vi "rqcAlice Cascade (Low Level Example).vi"() -> ()   [LabVIEW 2019]
panel:
  out "?":T1
  in  "QBER":dbl
  in  "Raw Alice's key path":string
  in  "Bob's port":string
  in  "Bob's IP":string
  out "pyton script path":path=path "../python_scripts/cascade_alice.py"
  in  "error in":errorcluster
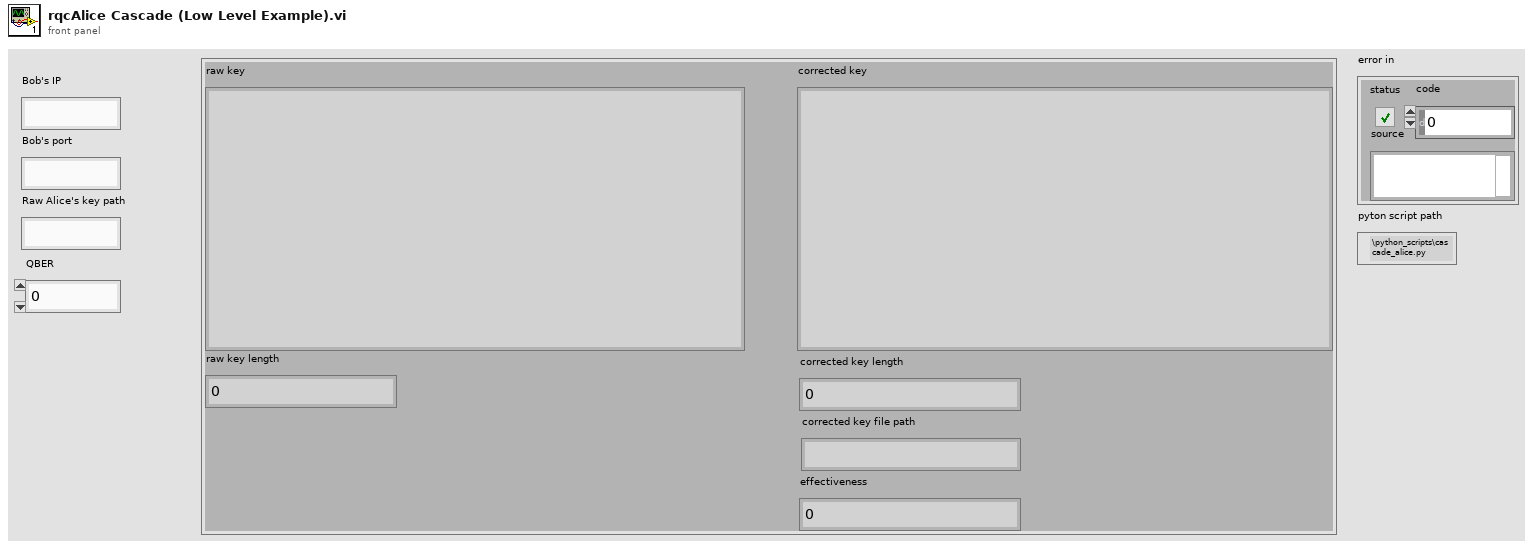
[diagram p1: front panel]
types:
  T1 = cluster{"raw key length":i32, "corrected key":string, "corrected key file path":string, "corrected key length":i32, "effectiveness":dbl, "raw key":string}
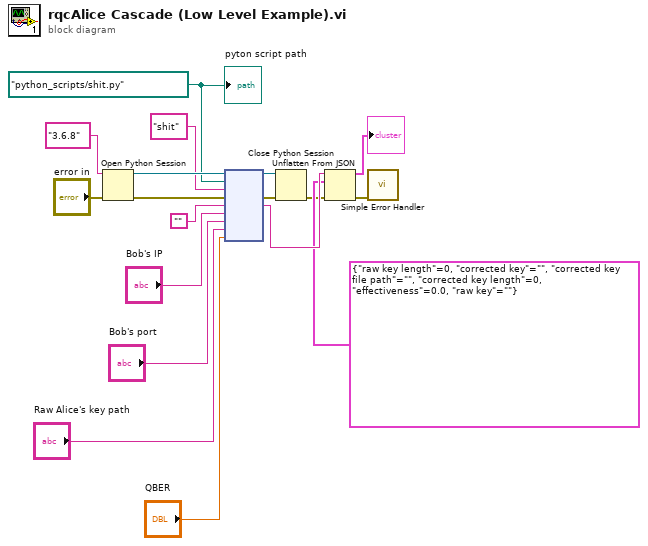
[diagram p0: block diagram]
diagram:
  w12 = path "python_scripts/shit.py" ("module path")
  n1 = Open Python Session(python version="3.6.8" ("Python version"), 3:"error in") -> (session out=w16:refnum<k35>, error out=w15:errorcluster)  [unwired: 1 in]
  n2 = node(w16, w12, "shit" ("function name"), w15, "", "Bob's IP", "Bob's port", "Raw Alice's key path", "QBER") -> (w14:refnum<k35>, w3:errorcluster, w7:string)  [unwired: 4 in, 2 out]
  n3 = Close Python Session(session in=w14, error in=w3) -> (11:w2:errorcluster)
  n4 = Unflatten From JSON(JSON string=w7, type and defaults=T1 {"raw key length"=0, "corrected key"="", "corrected key file path"="", "corrected key length"=0, "effectiveness"=0.0, "raw key"=""}, error in (no error)=w2) -> (value=→"?":T1, error out=w1:errorcluster)  [unwired: 4 in]
  n5 = call <vilib>:"Simple Error Handler.vi"("error in (no error)"=w1) -> ()  [unwired: 4 in, 5 out]
  "pyton script path" <- w12
